vi "Connecting(Sub VI).vi"() -> ()   [LabVIEW 2017]
uses:
  st_voltmetr/subVIs/st_str Global.vi
panel:
  in  "Boolean":bool
  out "String":string="Подключение."
  out "Slide":cluster{u8, u8}(slide)={0, 81} scale=0.0..100.0
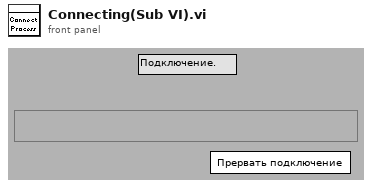
[diagram p1: front panel]
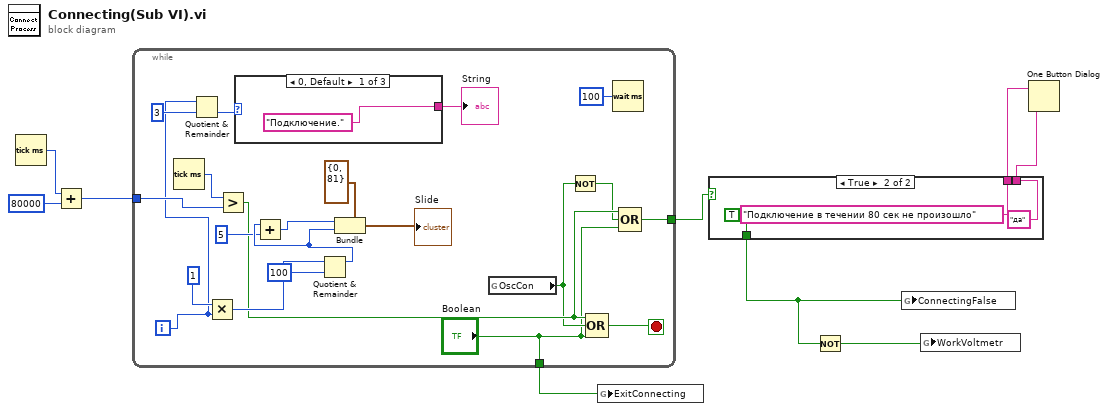
[diagram p0: block diagram]
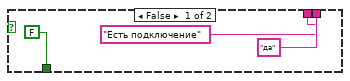
[diagram p2: hidden frame]
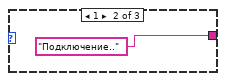
[diagram p3: hidden frame]
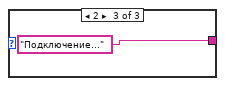
[diagram p4: hidden frame]
diagram:
  n1 = Tick Count (ms)() -> (millisecond timer value=w9:u32)
  n2 = Add(x=w9, y=u32 80000) -> (x+y=w7:u32)
  n3 = while {
    tunnel: w7 -> [w27]
    tunnel: [w13] -> w4
    tunnel: ["Boolean"] -> w3
    i -> [w22]
    stop <- w15 stop-if-true
    n4 = Tick Count (ms)() -> (millisecond timer value=w28:u32)
    n5 = Quotient & Remainder(x=w22, y=3) -> (floor(x/y)=w21:i32)  [unwired: 1 out]
    n6 = Multiply(x=1, y=w22) -> (x*y=w24:i32)
    n7 = Greater?(x=w28, y=w27) -> (0:w14:bool)
    n8 = case shown="0, Default" w21 {
      tunnel: ["Подключение." ("String") "Подключение.." ("String") "Подключение..." ("String")] -> w29
      frame 0, Default {
      }
      frame 1 {
      }
      frame 2 {
      }
    }
    "String" <- w29
    n9 = Quotient & Remainder(x=w24, y=100) -> (x-y*floor(x/y)=w18:i32)  [unwired: 1 out]
    n10 = Add(x=w18, y=5) -> (x+y=w16:i32)
    n11 = Bundle(cluster=cluster{u8, u8} {0, 81} ("Slide"), w16, w18) -> (→"Slide":cluster{u8, u8})
    n12 = global read "st_str Global.vi" "OscCon"() -> (w12:bool)
    n13 = Not(x=w12) -> (.not. x?=w11:bool)
    n14 = Compound Arithmetic op=OR(w14, w12, "Boolean") -> (w15:bool)
    n15 = Wait (ms)(milliseconds to wait=u32 100) -> ()  [unwired: 1 out]
    n16 = Compound Arithmetic op=OR(w14, w11, "Boolean") -> (w13:bool)
  }
  n17 = global write "st_str Global.vi" "ExitConnecting"(w3) -> ()
  n18 = case shown="True" w4 {
    tunnel: ["да" ("button name (\"OK\")") "да" ("button name (\"OK\")")] -> w5
    tunnel: ["Есть подключение" ("message") "Подключение в течении 80 сек не произошло" ("message")] -> w6
    tunnel: [FALSE ("ConnectingFalse") TRUE ("ConnectingFalse")] -> w2
    frame False {
    }
    frame True {
    }
  }
  n19 = Not(x=w2) -> (.not. x?=w1:bool)
  n20 = global write "st_str Global.vi" "ConnectingFalse"(w2) -> ()
  n21 = global write "st_str Global.vi" "WorkVoltmetr"(w1) -> ()
  n22 = One Button Dialog(message=w6, button name ("OK")=w5) -> ()  [unwired: 1 out]
